vi "4Digit File Incrementer tmp.vi"(10 "Number":i32, 11 "path":path) -> (3 "appended path":path)   [LabVIEW 2014]
panel:
  out "name 2":string
  out "before substring":string
  in  "error in (no error)":errorcluster
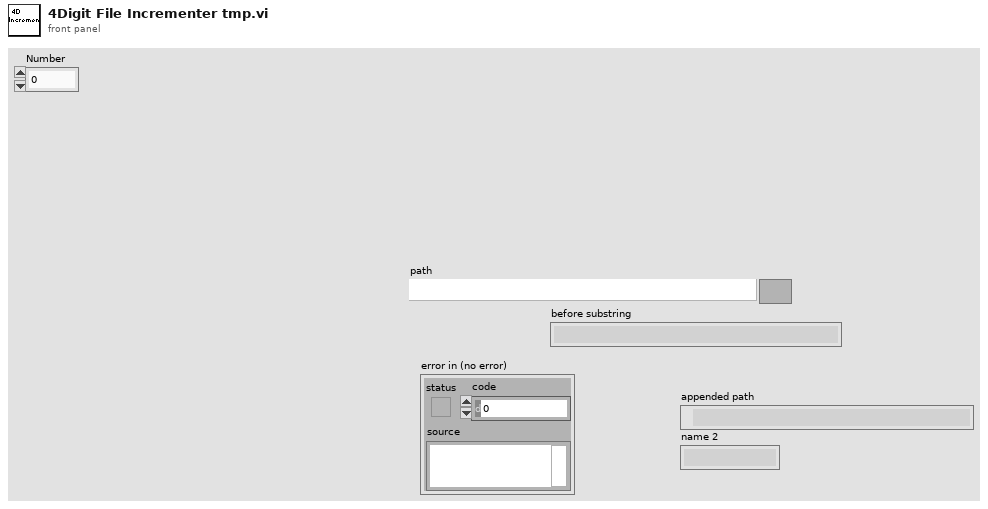
[diagram p1: front panel]
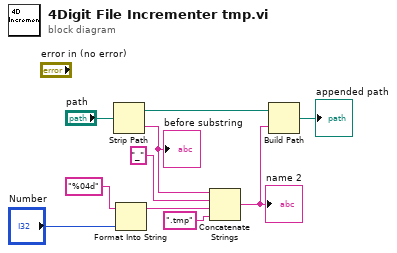
[diagram p0: block diagram]
diagram:
  n1 = Strip Path(path="path") -> (stripped path=w8:path, name=w6:string)
  "before substring" <- w6
  n2 = Format Into String(format string="%04d", "Number") -> (resulting string=w3:string)  [unwired: 2 in, 1 out]
  n3 = Concatenate Strings(w6, "_" ("string"), w3, ".tmp" ("string")) -> (w7:string)
  "name 2" <- w7
  n4 = Build Path(base path=w8, name or relative path=w7) -> (appended path=→"appended path":path)
